vi "Get Measure Configuration List Settings.vi"(0 "VISA resource name":refnum<visa-resource-name>, 1 "Configuration List Name":string, 2 "Configuration Point index (1)":u32=1, 3 "Specify Seperator Character (T:Yes)":bool=TRUE, 4 "Separator Character (0: Comma)":u16(ring) items=["Comma", "Semicolon", "New line"], 5 "error in (no error)":errorcluster) -> (14 "VISA resource name out":refnum<visa-resource-name>, 15 "Measure Configuration List settings":string, 19 "error out":errorcluster)   [LabVIEW 2020, in "Keithley 2450.lvlib"]
doc: "Returns a list of TSP commands that represent the parameters that are stored in the specified measure configuration list point."
uses:
  Keithley 2450.lvlib
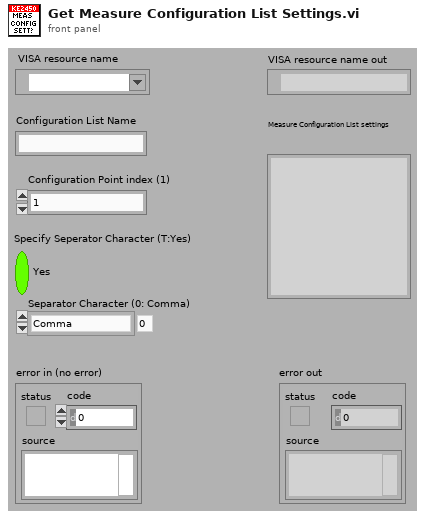
[diagram p1: front panel]
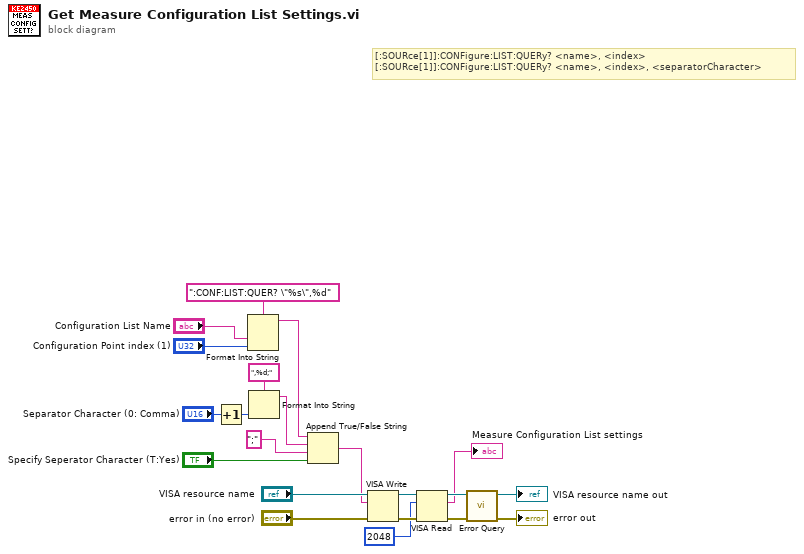
[diagram p0: block diagram]
diagram:
  # "[:SOURce[1]]:CONFigure:LIST:QUERy? <name>, <index>\n[:SOURce[1]]:CONFigure:LIST:QUERy? <name>, <index>, <separatorCharacter>"
  n1 = Increment(x="Separator Character (0: Comma)") -> (x+1=w11:u16)
  n2 = Format Into String(format string=":CONF:LIST:QUER? \"%s\",%d", "Configuration List Name", "Configuration Point index (1)") -> (resulting string=w7:string)  [unwired: 2 in, 1 out]
  n3 = Format Into String(format string=",%d;", w11) -> (resulting string=w14:string)  [unwired: 2 in, 1 out]
  n4 = Append True/False String(1:"Specify Seperator Character (T:Yes)", 2:";" ("false string"), 3:w14, 4:w7) -> (0:w9:string)
  n5 = VISA Write(VISA resource name="VISA resource name", write buffer=w9, error in (no error)="error in (no error)") -> (VISA resource name out=w6:refnum<visa-resource-name>, error out=w4:errorcluster)  [unwired: 1 out]
  n6 = VISA Read(VISA resource name=w6, byte count=u32 2048, error in (no error)=w4) -> (VISA resource name out=w5:refnum<visa-resource-name>, read buffer=→"Measure Configuration List settings":string, error out=w3:errorcluster)  [unwired: 1 out]
  n7 = call "Error Query.vi"("error in (no error)"=w3, "VISA resource name"=w5) -> ("error out"=→"error out":errorcluster, "VISA resource name out"=→"VISA resource name out":refnum<visa-resource-name>)  [unwired: 8 out]
